vi "Initialize.vi"(8 "error in (no error)":errorcluster, 11 "NHRDCModel in":refnum<class "NHRDCPowerModel.lvclass">) -> (0 "error out":errorcluster, 3 "NHRDCModel out":refnum<class "NHRDCPowerModel.lvclass">)   [LabVIEW 2018, in "AcPwrPlugins.lvlib" / "NHRDCPowerModel.lvclass"]
doc: "This VI establishes communication to the instrument and may provide other functions such as reset the instrument or provide a range check."
uses:
  NHRDCPowerModel.lvclass
  Database/DatabaseBaseClass/DatabaseBaseClass.lvclass
  TypeDefs/NHRDC__ICDAS2Model.ctl
  TypeDefs/NHRDC_Model2ICDAS.ctl
  NHRDCPowerModel.lvclass/NHRDCPowerModel.ctl
  <vilib>/addons/database/NI_Database_API.lvlib
  AcPwrBaseClass/AcPwrBase.lvclass
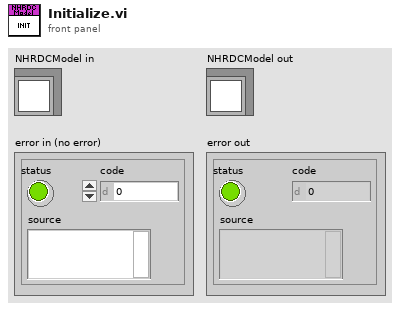
[diagram p1: front panel]
types:
  T1 = typedef "AcPwrPlugins.lvlib/NHRDCPowerModel.lvclass/NHRDC_Model2ICDAS.ctl" = cluster{"data_id":i32, "voltage":dbl, "current":dbl, "power":dbl, "meas_timestamp":timestamp, "write_timestamp":timestamp, "read_by_icdas":bool, "read_timestamp":timestamp}
  T2 = typedef "AcPwrPlugins.lvlib/NHRDCPowerModel.lvclass/NHRDC__ICDAS2Model.ctl" = cluster{"data_id":i32, "operating_state":i32, "Voltage":dbl, "Current":dbl, "Resistance":dbl, "Power":dbl, "Voltage_Slew_Rate":dbl, "Current_Slew_Rate":dbl, "Resistance_Slew_Rate":dbl, "Power_Slew_Rate ":dbl, "Battery_Detect_Voltage":dbl, "Max_Voltage_Time":dbl, "Max_Current":dbl, "Max_Current_Time":dbl, "Max_Power":dbl, "Max_Power_Time":dbl, "Max_Voltage":dbl, "write_timestamp":timestamp, "read_by_model":bool, "read_timestamp":timestamp, "meas_interval_ms":u32}
  T3 = typedef "AcPwrPlugins.lvlib/NHRDCPower.lvclass/Measurements.ctl" = cluster{"Handle":string, "Name":string, "Enabled":bool, "Measurement Value":sgl, "Measurement Type":enum16{"Power", "Current", "Voltage"}}[]
  T4 = typedef "AcPwrPlugins.lvlib/NHRDCPower.lvclass/Device(s)Settings.ctl" = cluster{"MeasName":string, "Modules":T5}
  T5 = typedef "AcPwrPlugins.lvlib/NHRDCPower.lvclass/Modules.ctl" = cluster{"Handle":string, "Name":string, "id query (Yes)":bool, "reset device (Yes)":bool, "Connected":bool, "Initial Battery Detect Voltage (0)":dbl, "SafetySettings":cluster{"SetWatchDog?":bool, "Voltage (V)":dbl, "Current (A)":dbl, "Power (W)":dbl, "Voltage Delay (s)":dbl, "Current Delay (s)":dbl, "Power Delay (s)":dbl}, "Options String":string, "Aperture Time (s)":dbl, "operating state (Off)":i32, "OutputSettings":cluster{"Voltage (V)":dbl, "Current (A)":dbl, "Resistance (Ohms)":dbl, "Power (W)":dbl, "Enable Voltage":bool, "Enable Current":bool, "Enable Resistance":bool, "Enable Power":bool, "Macro After Step Delay  (s)":dbl, "Wait Value (V, A, W)":dbl, "Enable Wait":bool, "Wait on Value":i32}, "SlewRate":cluster{"Set Voltage Rate V/S":dbl, "Set Current Rate A/S":dbl, "Set Resistance Rate R/S":dbl, "Set Power Rate W/S":dbl}, "Macro":cluster{"Save Macro?":bool, "Load Macro From File?":bool, "Run Macro Continuously?":bool, "Use Macros?":bool, "Load Macro File Path":path, "Save Macro File Path":string}, "Regulation Gain (1=100%)":dbl, "UpdatingOntheFly":bool}[]
  T6 = typedef "AcPwrShared.lvlib/Database Settings.ctl" = cluster{"Data Source":string, "ICDAS to Model Table":string, "Model to ICDAS Table":string}
  T7 = typedef "NI_Database_API.lvlib/Conn ObjectReference.ctl" = refnum<k1>
  T8 = cluster{"Handle":string, "Name":string, "id query (Yes)":bool, "reset device (Yes)":bool, "Connected":bool, "Initial Battery Detect Voltage (0)":dbl, "SafetySettings":cluster{"SetWatchDog?":bool, "Voltage (V)":dbl, "Current (A)":dbl, "Power (W)":dbl, "Voltage Delay (s)":dbl, "Current Delay (s)":dbl, "Power Delay (s)":dbl}, "Options String":string, "Aperture Time (s)":dbl, "operating state (Off)":i32, "OutputSettings":cluster{"Voltage (V)":dbl, "Current (A)":dbl, "Resistance (Ohms)":dbl, "Power (W)":dbl, "Enable Voltage":bool, "Enable Current":bool, "Enable Resistance":bool, "Enable Power":bool, "Macro After Step Delay  (s)":dbl, "Wait Value (V, A, W)":dbl, "Enable Wait":bool, "Wait on Value":i32}, "SlewRate":cluster{"Set Voltage Rate V/S":dbl, "Set Current Rate A/S":dbl, "Set Resistance Rate R/S":dbl, "Set Power Rate W/S":dbl}, "Macro":cluster{"Save Macro?":bool, "Load Macro From File?":bool, "Run Macro Continuously?":bool, "Use Macros?":bool, "Load Macro File Path":path, "Save Macro File Path":string}, "Regulation Gain (1=100%)":dbl, "UpdatingOntheFly":bool}
  T9 = cluster{"Device(s)Settings":T4, "Database Settings":T6}
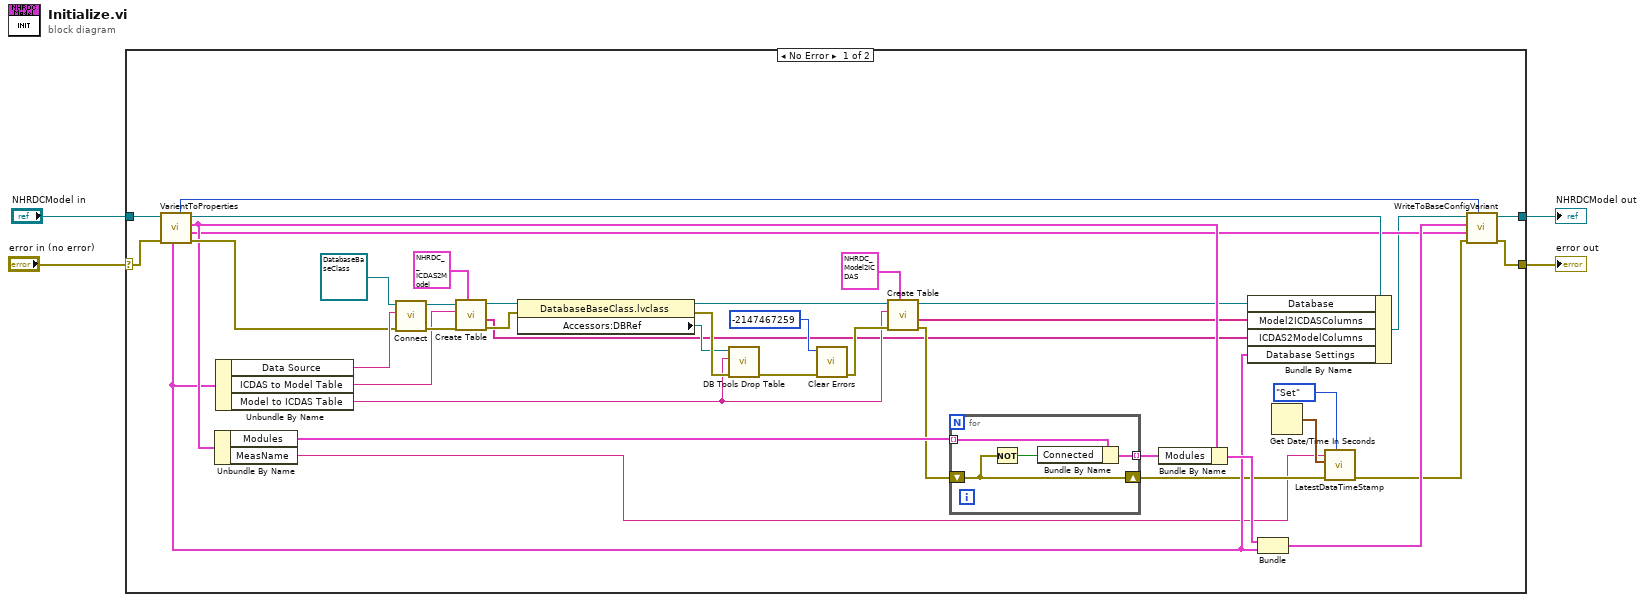
[diagram p0: block diagram]
diagram:
  n1 = case shown="No Error" "error in (no error)" {
    selector: "error in (no error)" -> [w43 w49]
    tunnel: "NHRDCModel in" -> [w44 w50]
    tunnel: [w6 w50] -> w2
    tunnel: [w39 w49] -> w1
    frame No Error {
      n2 = call "VarientToProperties.vi"("error in (no error)"=w43, "AcPwrPlugins.lvlib:NHRDCModel.lvclass"=w44) -> ("error out"=w40:errorcluster, "Measurements"=w8:T3, "Device(s)Settings"=w22:T4, "AcPwrPlugins.lvlib:NHRDCModel.lvclass"=w18:refnum<class "NHRDCPowerModel.lvclass">, "Measurement Refresh Time (ms)"=w5:u32, "Database Settings"=w14:T6)  [unwired: 4 in]
      n3 = Unbundle By Name(w22) -> ("Modules"=w24:T5, "MeasName"=w11:string)
      n4 = Unbundle By Name(w14) -> ("Data Source"=w41:string, "ICDAS to Model Table"=w36:string, "Model to ICDAS Table"=w26:string)
      n5 = call-dynamic "Connect.vi"("error in (no error)"=w40, "Data Source"=w41, "DatabaseBaseClass in"=refnum<class "DatabaseBaseClass.lvclass"> refnum) -> ("error out"=w38:errorcluster, "DatabaseBaseClass out"=w37:refnum<class "DatabaseBaseClass.lvclass">)  [unwired: 7 in]
      n6 = call-dynamic "Create Table.vi"("Cluster In"=T2 {"data_id"=0, "operating_state"=0, "Voltage"=0.0, "Current"=0.0, "Resistance"=0.0, "Power"=0.0, "Voltage_Slew_Rate"=0.0, "Current_Slew_Rate"=0.0, "Resistance_Slew_Rate"=0.0, "Power_Slew_Rate "=0.0, "Battery_Detect_Voltage"=0.0, "Max_Voltage_Time"=0.0, "Max_Current"=0.0, "Max_Current_Time"=0.0, "Max_Power"=0.0, "Max_Power_Time"=0.0, "Max_Voltage"=0.0, "write_timestamp"=timestamp(0 s since 1904-01-01), "read_by_model"=FALSE, "read_timestamp"=timestamp(0 s since 1904-01-01), "meas_interval_ms"=0} ("NHRDC_ICDAS2Model"), "error in (no error)"=w38, "Table Name"=w36, "DatabaseBaseClass In"=w37) -> ("error out"=w33:errorcluster, "Column Names"=w15:string[], "DatabaseBaseClass out"=w34:refnum<class "DatabaseBaseClass.lvclass">)  [unwired: 4 in, 1 out]
      n7 = property class="DatabaseBaseClass.lvclass"(reference=w34, error in=w33) -> (reference out=w28:refnum<class "DatabaseBaseClass.lvclass">, error out=w30:errorcluster, "Accessors:DBRef"=w29:T7)
      n8 = call <vilib>:"DB Tools Drop Table.vi"("error in (no error)"=w30, "table"=w26, "connection reference"=w29) -> ("error out"=w32:errorcluster)  [unwired: 5 in, 1 out]
      n9 = call <vilib>:"Clear Errors.vi"("error in (no error)"=w32, "specific error code to clear (0: all)"=-2147467259) -> ("error out"=w27:errorcluster)  [unwired: 4 in, 1 out]
      n10 = call-dynamic "Create Table.vi"("Cluster In"=T1 {"data_id"=0, "voltage"=0.0, "current"=0.0, "power"=0.0, "meas_timestamp"=timestamp(0 s since 1904-01-01), "write_timestamp"=timestamp(0 s since 1904-01-01), "read_by_icdas"=FALSE, "read_timestamp"=timestamp(0 s since 1904-01-01)} ("NHRDC_Model2ICDAS"), "error in (no error)"=w27, "Table Name"=w26, "DatabaseBaseClass In"=w28) -> ("error out"=w23:errorcluster, "Column Names"=w16:string[], "DatabaseBaseClass out"=w17:refnum<class "DatabaseBaseClass.lvclass">)  [unwired: 4 in, 1 out]
      n11 = for {
        tunnel: w24 -> [w48] mode=indexing
        shift-right: [w46] -> w13
        shift-left: w23 -> [w46]
        tunnel: [w47] -> w21 mode=indexing
        n12 = Not(x=w46) -> (.not. x?=w45:bool)
        n13 = Bundle By Name(cluster=w48, "Connected"=w45) -> (w47:T8)
      }
      n14 = Bundle By Name(cluster=w22, "Modules"=w21) -> (w20:T4)
      n15 = Bundle By Name(cluster=w18, "Database"=w17, "Model2ICDASColumns"=w16, "ICDAS2ModelColumns"=w15, "Database Settings"=w14) -> (w7:refnum<class "NHRDCPowerModel.lvclass">)
      n16 = Bundle("Device(s)Settings"=w20, "Database Settings"=w14) -> (w19:T9)  [unwired: 1 in]
      n17 = Get Date/Time In Seconds() -> (seconds since 1Jan1904=w12:timestamp)
      n18 = call "LatestDataTimeStamp.vi"("Action"=enum16{"Set", "Get"}."Set", "error in (no error)"=w13, "TimeStamp"=w12, "Plugin Name"=w11) -> ("error IO"=w9:errorcluster)  [unwired: 5 in, 2 out]
      n19 = call-dynamic "WriteToBaseConfigVariant.vi"("Measurement Refresh Time (ms)"=w5, "error in (no error)"=w9, "Meas"=w8, "Config"=w19, "NHRDCModel in"=w7) -> ("error out"=w39:errorcluster, "NHRDCModel out"=w6:refnum<class "NHRDCPowerModel.lvclass">)  [unwired: 5 in]
    }
    frame Error {
    }
  }
  "error out" <- w1
  "NHRDCModel out" <- w2
